vi "Unix time string to time stamp.vi"(5 "Unix time string [ms]":string) -> (2 "Time stamp":timestamp)   [LabVIEW 2025]
doc: "Converts a UNIX based time string in ms into a LabVIEW based time stamp."
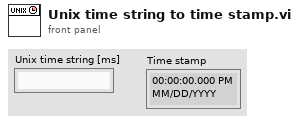
[diagram p1: front panel]
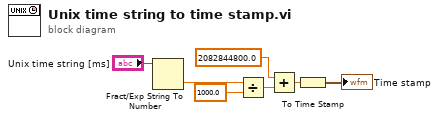
[diagram p0: block diagram]
diagram:
  n1 = Fract/Exp String To Number(string="Unix time string [ms]") -> (number=w5:dbl)  [unwired: 3 in, 1 out]
  n2 = Divide(x=w5, y=1000.0) -> (x/y=w4:dbl)
  n3 = Add(x=2082844800.0, y=w4) -> (x+y=w6:dbl)
  n4 = To Time Stamp(1:w6) -> (0:→"Time stamp":timestamp)
